vi "Change Label Style.vi"(8 "error in":errorcluster, 10 "Settinngs":T1, 11 "VI in":refnum<vi>) -> (0 "error out":errorcluster, 3 "VI out":refnum<vi>)   [LabVIEW 2019]
uses:
  <vilib>/Utility/traverseref.llb/VI Scripting - Traverse.lvlib
  <vilib>/Utility/traverseref.llb/TRef TravTarget.ctl
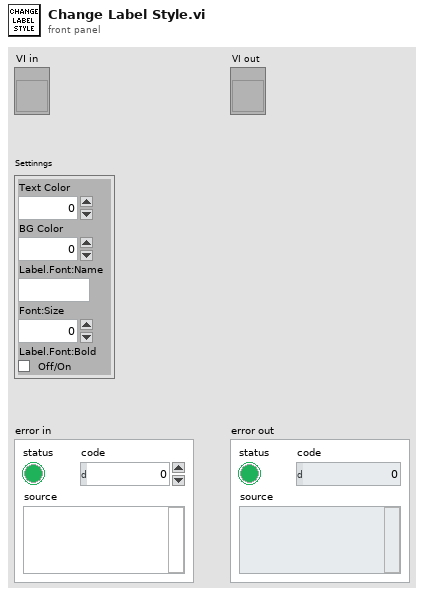
[diagram p1: front panel]
types:
  T1 = cluster{"Text Color":u32, "BG Color":u32, "Label.Font:Name":string, "Font:Size":u32, "Label.Font:Bold":bool}
  T2 = typedef "TRef TravTarget.ctl" = enum16{"FP", "BD", "Other"}
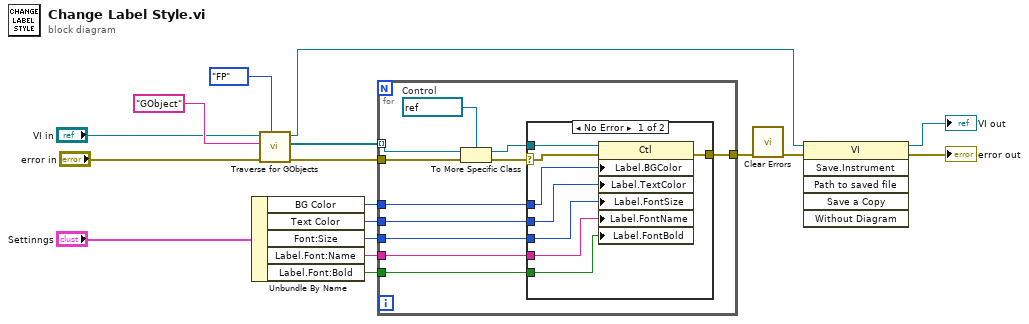
[diagram p0: block diagram]
diagram:
  n1 = Unbundle By Name("Settinngs") -> ("BG Color"=w5:u32, "Text Color"=w4:u32, "Font:Size"=w3:u32, "Label.Font:Name"=w2:string, "Label.Font:Bold"=w1:bool)
  n2 = call <vilib>:"Traverse for GObjects.vi"("Traverse Target"=TRef_TravTarget."FP", "error in (no error)"="error in", "Class Name"="GObject", "VI Refnum"="VI in") -> ("error out"=w15:errorcluster, "References"=w10:refnum<vi>[], "dup VI Refnum"=w11:refnum<vi>)  [unwired: 4 in, 1 out]
  n3 = for {
    tunnel: w10 -> [w25] mode=indexing
    tunnel: w15 -> [w27]
    tunnel: w5 -> [w22]
    tunnel: [w26] -> w16
    tunnel: w4 -> [w21]
    tunnel: w3 -> [w20]
    tunnel: w2 -> [w19]
    tunnel: w1 -> [w18]
    w24 = refnum<vi> refnum  # Control
    n4 = To More Specific Class(target class=w24, reference=w25, error in=w27) -> (specific class reference=w23:refnum<vi>, error out=w28:errorcluster)
    n5 = case shown="No Error" w28 {
      selector: w28 -> [w36 w37]
      tunnel: w23 -> [w34 _]
      tunnel: w22 -> [w33 _]
      tunnel: [w35 w37] -> w26
      tunnel: w21 -> [w32 _]
      tunnel: w20 -> [w31 _]
      tunnel: w19 -> [w30 _]
      tunnel: w18 -> [w29 _]
      frame No Error {
        n6 = property class="Ctl"(reference=w34, error in=w36, "Label.BGColor"=w33, "Label.TextColor"=w32, "Label.FontSize"=w31, "Label.FontName"=w30, "Label.FontBold"=w29) -> (error out=w35:errorcluster)  [unwired: 1 out]
      }
      frame Error {
      }
    }
  }
  n7 = call <vilib>:"Clear Errors.vi"("error in (no error)"=w16) -> ("error out"=w17:errorcluster)  [unwired: 5 in, 1 out]
  n8 = invoke class="VI" method="Save.Instrument"(reference=w11, error in=w17) -> (reference out=→"VI out":refnum<vi>, error out=→"error out":errorcluster)  [unwired: 4 in, 4 out]
